vi "WPI_CameraAcquire Image.vi"(11 "Camera Address":string) -> ()   [LabVIEW 2017]
doc: "This VI is the image pump. It acquires images as long as somebody needs it. \n\nThis software is licensed. Open the labview\\readme\\WPI Robotics Library Open Source License.txt file for more information."
uses:
  <vilib>/Rock Robotics/WPI/Camera/WPI_CameraFrameRate.ctl
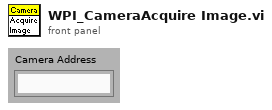
[diagram p1: front panel]
types:
  T1 = typedef "WPI_CameraFrameRate.ctl" = u32
  T2 = typedef "Camera.lvlib/FrameRate.ctl" = u32
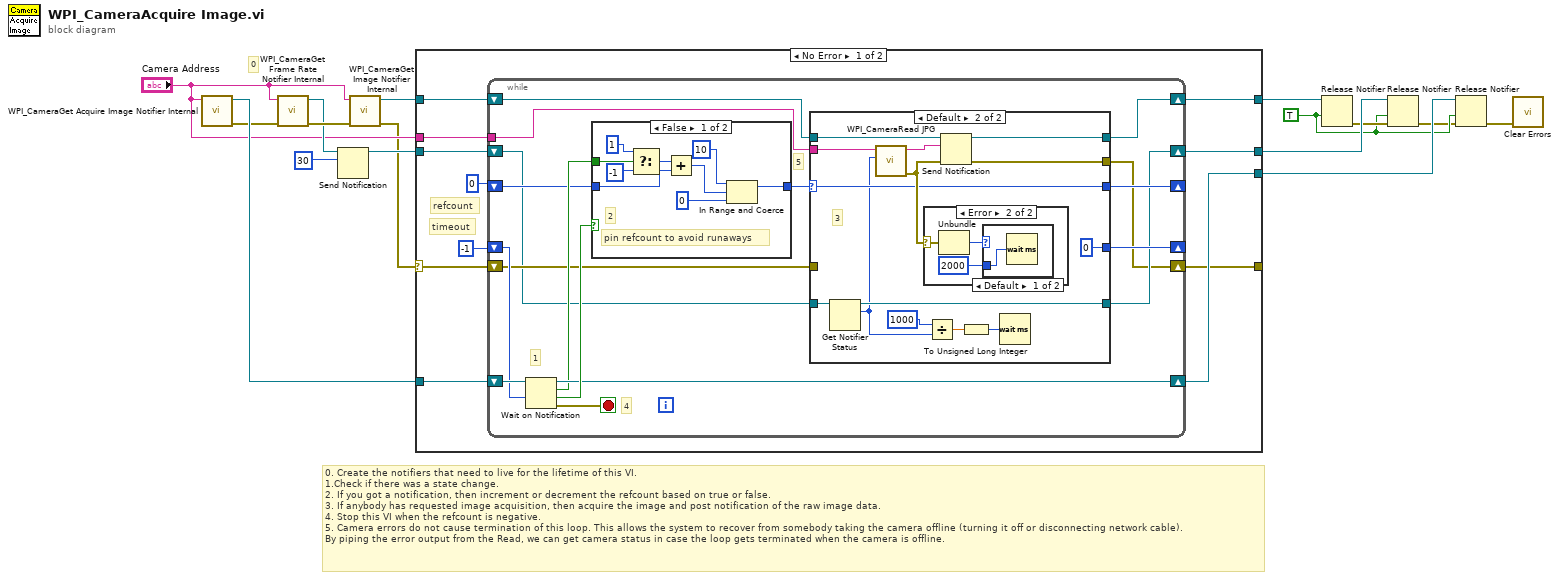
[diagram p0: block diagram]
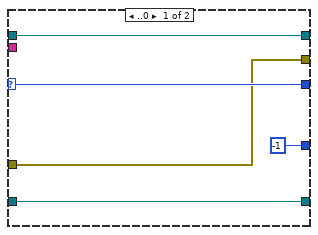
[diagram p2: hidden frame]
diagram:
  w7 = TRUE ("force destroy? (F)")
  # "0"
  # "0. Create the notifiers that need to live for the lifetime of this VI. \n1.Check if there was a state change.\n2. If you got a notification, then increment or decrement the refcount based on true or false.\n3. If anybody has requested image acquisition, then acquire the image and post notification of the raw image data.\n4. Stop this VI when the refcount is negative.\n5. Camera errors do not cause termination of this loop. This allows the system to recover from somebody taking the camera offline (turning it off or disconnecting network cable).\nBy piping the error output from the Read, we can get camera status in case the loop gets terminated when the camera is offline."
  n1 = call <vilib>:"WPI_CameraGet Acquire Image Notifier Internal.vi"("Camera Address"="Camera Address") -> ("error out"=w6:errorcluster, "Acquire Image Notifier"=w14:refnum<notifier>)  [unwired: 1 in, 8 out]
  n2 = call <vilib>:"WPI_CameraGet Frame Rate Notifier Internal.vi"("error in (no error)"=w6, "Camera Address"="Camera Address") -> ("error out"=w12:errorcluster, "Image Rate Notifier"=w11:refnum<notifier>)  [unwired: 8 out]
  n3 = Send Notification(notification=T1 30 ("Frame Rate (fps)"), notifier=w11) -> (notifier out=w10:refnum<notifier>)  [unwired: 1 in, 1 out]
  n4 = call <vilib>:"WPI_CameraGet Image Notifier Internal.vi"("error in (no error)"=w12, "Camera Address"="Camera Address") -> ("error out"=w3:errorcluster, "Image Notifier"=w13:refnum<notifier>)  [unwired: 8 out]
  n5 = case shown="No Error" w3 {
    selector: w3 -> [w20 w81]
    tunnel: "Camera Address" -> [w27 _]
    tunnel: w14 -> [w26 w79]
    tunnel: w13 -> [w24 w80]
    tunnel: [w22 w80] -> w16
    tunnel: [w21 w79] -> w15
    tunnel: [w19 w81] -> _
    tunnel: w10 -> [w18 w78]
    tunnel: [w17 w78] -> w9
    frame No Error {
      # "timeout"
      # "refcount"
      n6 = while {
        shift-right: [w42] -> w21
        shift-left: w26 -> [w44]
        tunnel: w27 -> [w39]
        shift-right: [w31] -> _
        shift-left: 0 -> [w40]
        shift-right: [w37] -> w22
        shift-left: w24 -> [w38]
        shift-right: [w35] -> _
        shift-left: -1 -> [w36]
        shift-right: [w28] -> w19
        shift-left: w20 -> [w33]
        shift-right: [w29] -> w17
        shift-left: w18 -> [w30]
        stop <- w34 stop-if-true
        # "5"
        # "4"
        # "1"
        n7 = Wait on Notification(notifier=w44, timeout in ms (-1)=w36) -> (notifier out=w42:refnum<notifier>, notification=w41:bool, timed out?=w43:bool, error out=w34:errorcluster)  [unwired: 1 in, 1 out]
        n8 = case shown="False" w43 {
          tunnel: w41 -> [w76 _]
          tunnel: w40 -> [w72 w77]
          tunnel: [w68 w77] -> w32
          frame False {
            # "pin refcount to avoid runaways"
            # "2"
            n9 = Select(t=1, s=w76, f=-1) -> (s? t:f=w73:i32)
            n10 = Add(x=w73, y=w72) -> (x+y=w69:i32)
            n11 = In Range and Coerce(upper limit=10, x=w69, lower limit=0) -> (coerced(x)=w68:i32)  [unwired: 1 out]
          }
          frame True {
          }
        }
        n12 = case shown="Default" w32 {
          selector: w32 -> [w48 w57]
          tunnel: w39 -> [_ w63]
          tunnel: w38 -> [w49 w62]
          tunnel: [w49 w61] -> w37
          tunnel: [-1 0] -> w35
          tunnel: w33 -> [w45 _]
          tunnel: [w48 w57] -> w31
          tunnel: w30 -> [w47 w53]
          tunnel: [w47 w52] -> w29
          tunnel: [w45 w50] -> w28
          frame ..0 {
          }
          frame Default {
            # "3"
            n13 = Get Notifier Status(notifier=w53) -> (notifier out=w52:refnum<notifier>, current notification=w51:T2)  [unwired: 1 in, 3 out]
            n14 = call <vilib>:"WPI_CameraRead JPG.vi"("fps"=w51, "address"=w63) -> ("error out"=w58:errorcluster, "Raw Image Data"=w59:string)  [unwired: 2 in, 6 out]
            n15 = case shown="Error" w58 {
              selector: w58 -> [_ w66]
              frame No Error {
              }
              frame Error {
                n16 = Unbundle(w66) -> ("code"=w65:i32)  [unwired: 2 out]
                n17 = case shown="Default" w65 {
                  tunnel: u32 2000 ("milliseconds to wait") -> [w67 _]
                  frame Default {
                    n18 = Wait (ms)(milliseconds to wait=w67) -> ()  [unwired: 1 out]
                  }
                  frame 56 {
                  }
                }
              }
            }
            n19 = Divide(x=T1 1000, y=w51) -> (x/y=w55:dbl)
            n20 = Send Notification(notification=w59, notifier=w62, error in (no error)=w58) -> (notifier out=w61:refnum<notifier>, error out=w50:errorcluster)
            n21 = To Unsigned Long Integer(number=w55) -> (unsigned 32bit integer=w56:u32)
            n22 = Wait (ms)(milliseconds to wait=w56) -> ()  [unwired: 1 out]
          }
        }
      }
    }
    frame Error {
    }
  }
  n23 = Release Notifier(notifier=w16, force destroy? (F)=w7) -> (error out=w8:errorcluster)  [unwired: 1 in, 2 out]
  n24 = Release Notifier(notifier=w9, force destroy? (F)=w7, error in (no error)=w8) -> (error out=w5:errorcluster)  [unwired: 2 out]
  n25 = Release Notifier(notifier=w15, force destroy? (F)=w7, error in (no error)=w5) -> (error out=w2:errorcluster)  [unwired: 2 out]
  n26 = call <vilib>:"Clear Errors.vi"("error in (no error)"=w2) -> ()  [unwired: 1 in, 6 out]
